vi "Read Connection String.vi"(4 "Error In":errorcluster, 7 "DB In":refnum<class "Config Data_DB.lvclass">) -> (0 "Error Out":errorcluster, 2 "Connection String":string, 3 "DB Out":refnum<class "Config Data_DB.lvclass">)   [LabVIEW 2014, in "Config Data.lvlib" / "Config Data_DB.lvclass"]
uses:
  Config Data_DB.lvclass
  Config Data_DB.lvclass/Config Data_DB.ctl
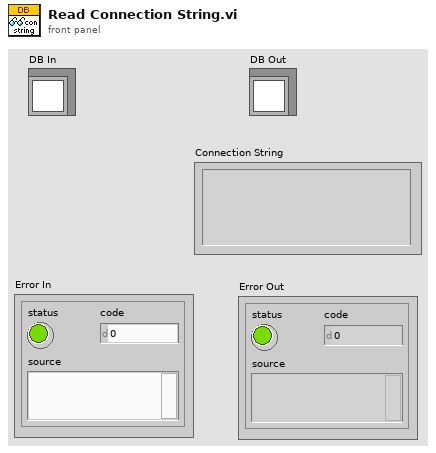
[diagram p1: front panel]
types:
  T1 = typedef "Config Data.lvlib/Config Data_DB.lvclass/DB Data.ctl" = cluster{"Connection String":string}
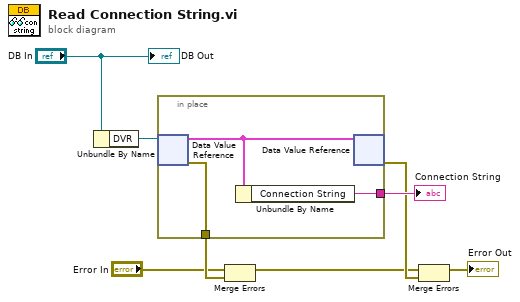
[diagram p0: block diagram]
diagram:
  n1 = Unbundle By Name("DB In") -> ("DVR"=w7:refnum<data-value>)
  n2 = in-place {
    in-place-border: [w11] -> w6
    in-place-border: [w9] -> w5
    n3 = in-place-dvr #1(w7) -> (w10:T1, w9:errorcluster)
    n4 = Unbundle By Name(w10) -> ("Connection String"=w11:string)
    n5 = in-place-dvr #1(w10) -> (w3:errorcluster)  [unwired: 1 out]
  }
  "Connection String" <- w6
  n6 = Merge Errors("Error In", w5) -> (w2:errorcluster)
  n7 = Merge Errors(w2, w3) -> (→"Error Out":errorcluster)
  "DB Out" <- "DB In"
